vi "Get Gas Output.vi"(8 "error in (no error)":errorcluster, 11 "Vapour Generator in":refnum<class "Vapour Generator.lvclass">) -> (0 "error out":errorcluster, 2 "Output":T1 {"Relative Humidity (%)" format="%#.4g"; "Flow Rate (ml/min)" format="%#.0f"; "Concentration (ppm)" format="%#.2g"}, 3 "Vapour Generator out":refnum<class "Vapour Generator.lvclass">)   [LabVIEW 2011, in "Vapour Generator.lvclass"]
uses:
  Vapour Generator.lvclass
  Gas Output.ctl
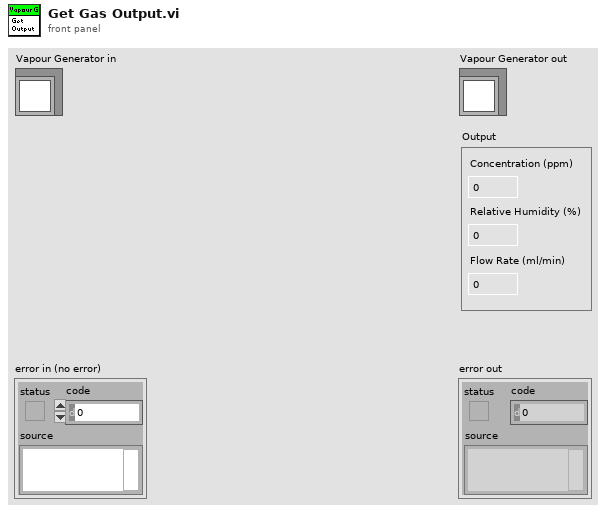
[diagram p1: front panel]
types:
  T1 = typedef "Vapour Generator.lvclass/Gas Output.ctl" = cluster{"Concentration (ppm)":dbl, "Flow Rate (ml/min)":dbl, "Relative Humidity (%)":dbl}
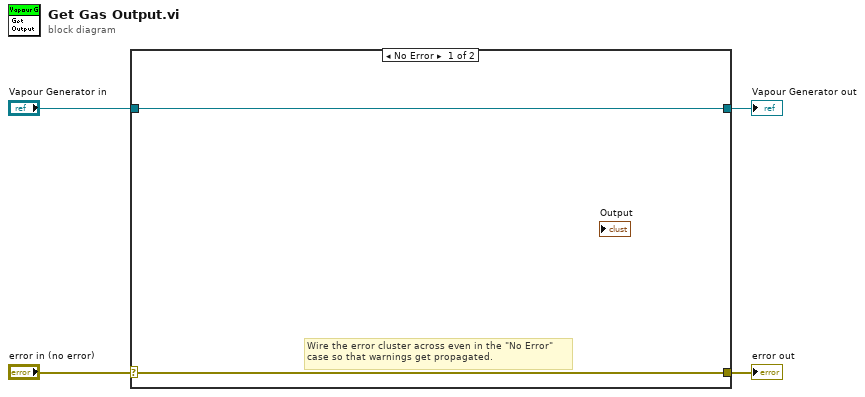
[diagram p0: block diagram]
diagram:
  n1 = case shown="No Error" "error in (no error)" {
    selector: "error in (no error)" -> [w5 w8]
    tunnel: [w5 w8] -> w3
    tunnel: [w6 w7] -> w1
    tunnel: "Vapour Generator in" -> [w6 w7]
    frame No Error {
      # "Wire the error cluster across even in the \"No Error\"\ncase so that warnings get propagated."
    }
    frame Error {
    }
  }
  "error out" <- w3
  "Vapour Generator out" <- w1
